vi "Constank Jerk Ref Mod (SubVI).vi"(0 "jav pos":dbl[](array[numeric])=[0.3, 0.2, 0.2], 1 "p_new":dbl[](array[numeric])=[2.0, 2.0, 0.0], 3 "Set point p":dbl[](array[numeric]), 4 "Eta":dbl[](array[numeric]), 5 "jav rad":dbl[](array[numeric])=[0.25, 0.15, 0.15], 7 "error in":errorcluster, 8 "Brake":bool, 9 "Set point theta":dbl[](array[numeric]), 10 "Go":bool, 12 "Go heading":bool, 13 "Theta_new":dbl[](array[numeric])=[0.0, 0.0, 45.0], 15 "time":dbl) -> (14 "javp":dbl[](array[numeric]), 16 "Eta des":dbl[](array[numeric]), 17 "Theta_ddot":dbl[](array[numeric]), 20 "Arrived":bool, 21 "Arrived yaw":bool, 23 "p_ddot":dbl[](array[numeric]), 24 "Nu des":dbl[](array[numeric]), 25 "Theta_d":dbl[](array[numeric]), 27 "error out":errorcluster)   [LabVIEW 2014, in "Guidance Library.lvlib" / "Constant Jerk Guidance.lvclass"]
uses:
  Constant Jerk Guidance.lvclass
  <vilib>/imath/engines/lvmath2/RunTimeEngine/BuiltInFunctions/rem/NIMS_rem_no checks.vi
  <instcachedir>/0/NIMS_rem_no checks_4BA74C9509D7485B8AB3E4C2ACC5A763.lvgen/NIMS_rem_no checks_4BA74C9509D7485B8AB3E4C2ACC5A763_000.vi
  <vilib>/imath/engines/lvmath2/RunTimeEngine/BuiltInFunctions/abs/NIMS_abs(signed).vi
  <instcachedir>/0/NIMS_abs(signed)_C4FCB8E6058B49B797C7C8D53CA5F6EC.lvgen/NIMS_abs(signed)_C4FCB8E6058B49B797C7C8D53CA5F6EC_000.vi
  <vilib>/imath/engines/lvmath2/RunTimeEngine/VariableToken/NIMS_VariableToken_CondDefined.vi
  <instcachedir>/0/NIMS_VariableToken_CondDefined_EE8DD211A89249938CE6537267F5C9B3.lvgen/NIMS_VariableToken_CondDefined_EE8DD211A89249938CE6537267F5C9B3_004.vi
  <vilib>/imathl/engines/lvmath/Functions/Error Handling/Create Error.vi
  <vilib>/imath/engines/lvmath2/RunTimeEngine/NodeEndStatement/NIMS_NodeEndStatement_Output.vi
  <instcachedir>/0/NIMS_NodeEndStatement_Output_53EC0D466D134D7ABD903AC30B43404B.lvgen/NIMS_NodeEndStatement_Output_53EC0D466D134D7ABD903AC30B43404B_001.vi
  <vilib>/imath/engines/lvmath2/RunTimeEngine/ErrorHandling/NIMS_Finalize Error.vi
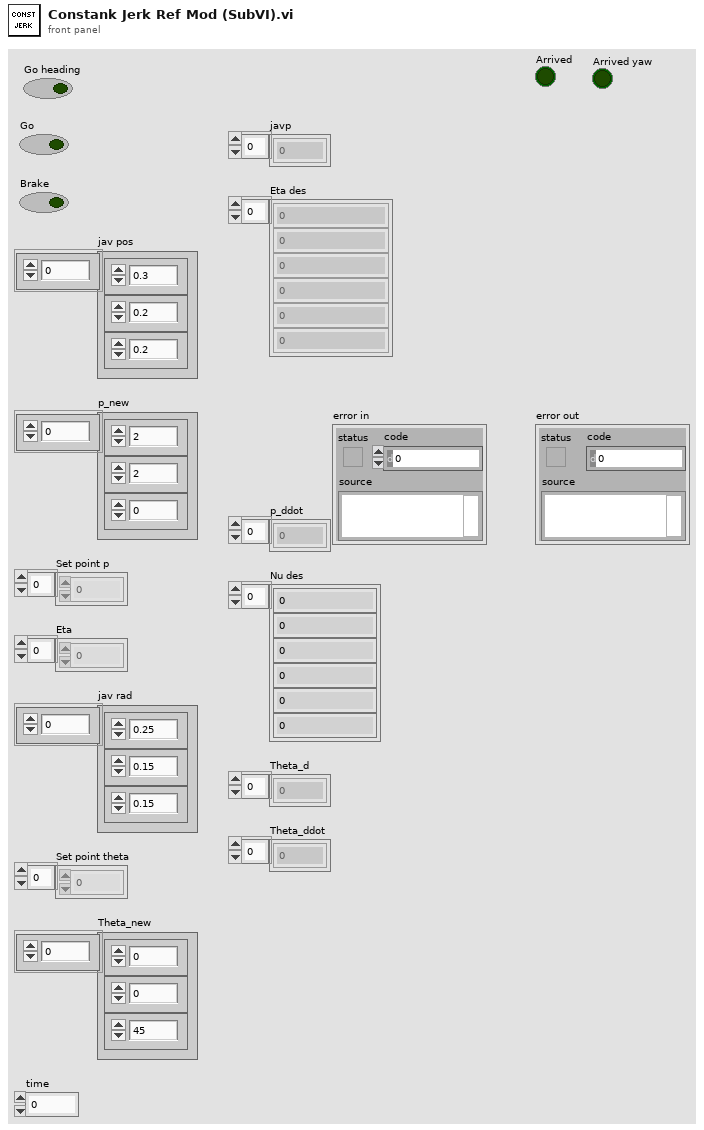
[diagram p1: front panel]
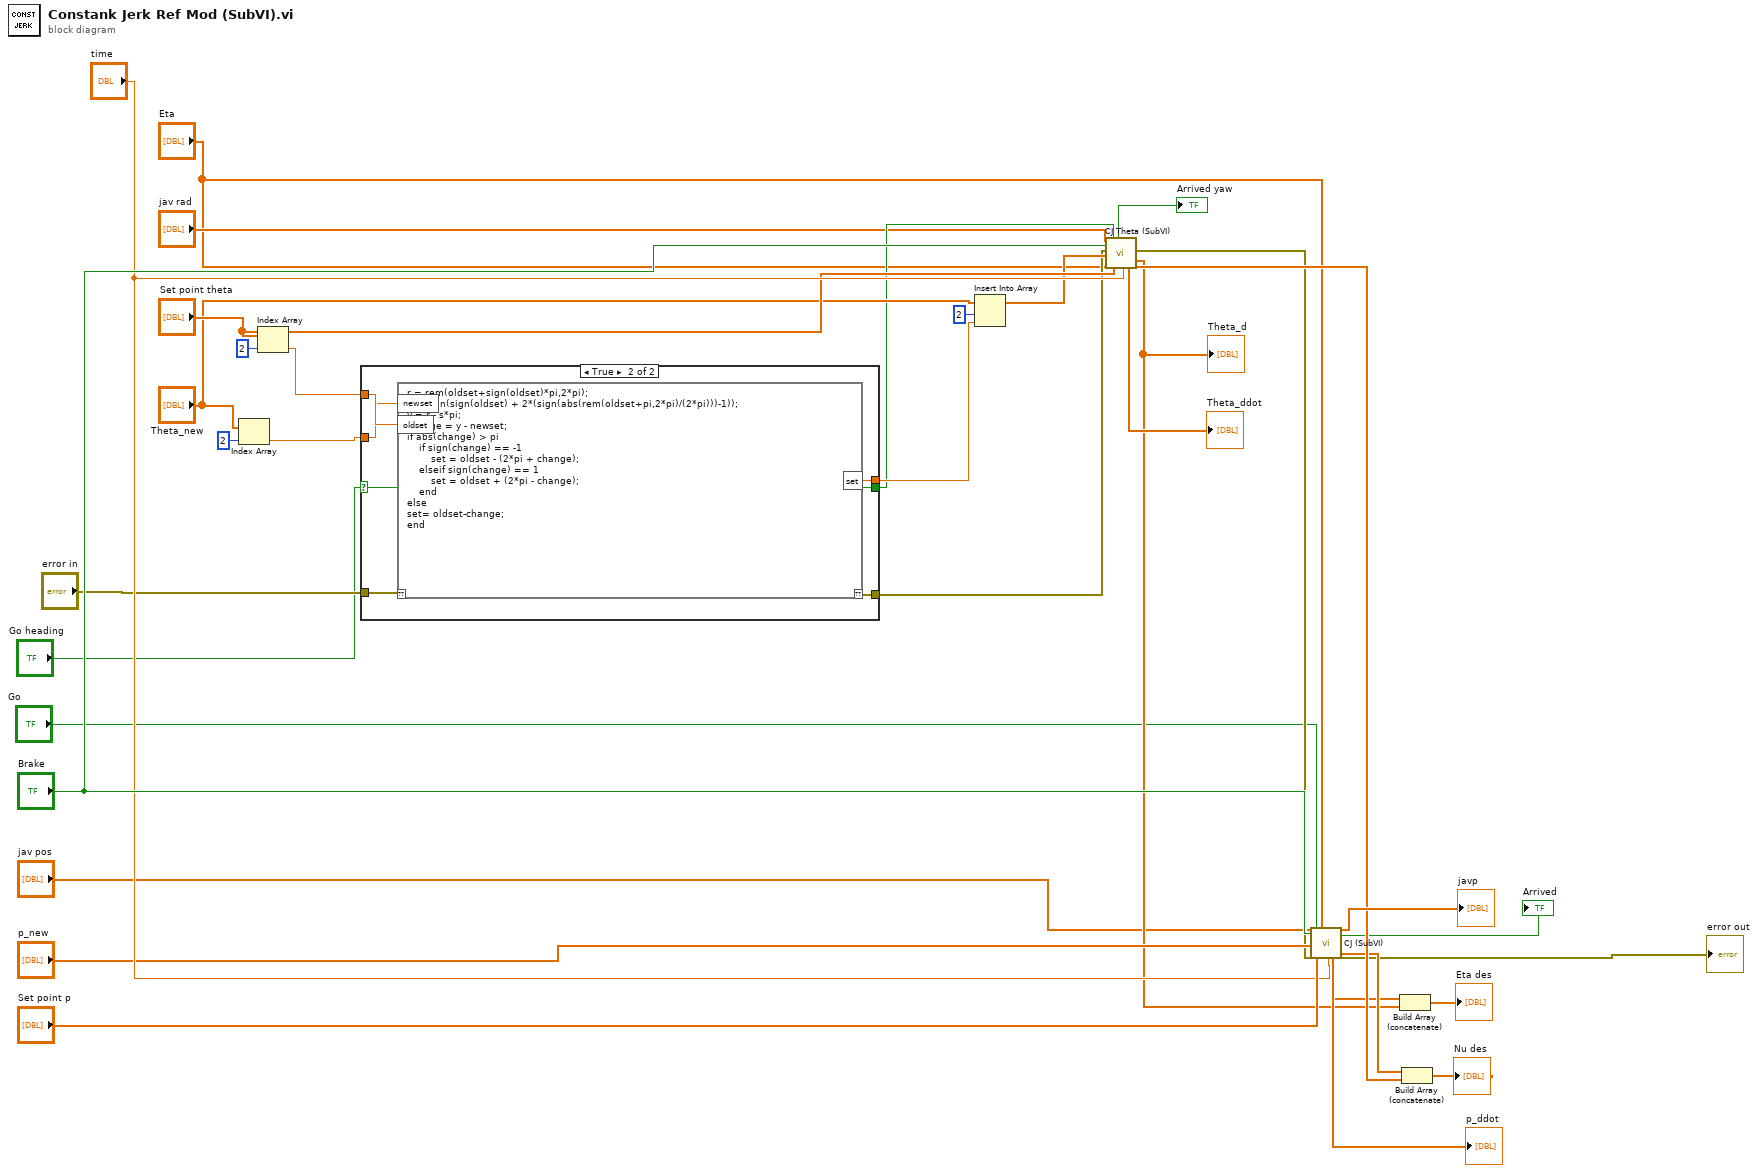
[diagram p0: block diagram]
diagram:
  n1 = Index Array(array="Theta_new", index=2) -> (element=w18:dbl)
  n2 = Index Array(array="Set point theta", index=2) -> (element=w20:dbl)
  n3 = case shown="True" "Go heading" {
    selector: "Go heading" -> [w35 w38]
    tunnel: w20 -> [_ w43]
    tunnel: w18 -> [w37 w42]
    tunnel: [w37 w41] -> w17
    tunnel: "error in" -> [w36 w40]
    tunnel: [w36 w39] -> w7
    tunnel: [w35 w38] -> w6
    frame False {
    }
    frame True {
      n4 = mathscript code="r = rem(oldset+sign(oldset)*pi,2*pi);\ns = sign(sign(oldset) + 2*(sign(abs(rem(oldset+pi,2*pi)/(2*pi)))-1));\ny = r - s*pi;\nchange = y - newset;\nif abs(change) > pi\n    if sign(change) == -1\n        set = oldset - (2*pi + change);\n    elseif sign(change) == 1\n        set = oldset + (2*pi - change);\n    end\nelse\nset= oldset-change;\nend"("??"=w40, "newset"=w42, "oldset"=w43) -> ("??"=w39:errorcluster, "set"=w41:dbl)
    }
  }
  n5 = Insert Into Array(array="Theta_new", index=2, new element=w17) -> (w14:dbl[])
  n6 = call "CJ Theta (SubVI).vi"("jav rad"="jav rad", "Brake"="Brake", "error in"=w7, "p_new"=w14, "Eta"="Eta", "Go"=w6, "p_old"="Set point theta", "time"="time") -> ("Arrived"=→"Arrived yaw":bool, "Theta_ddot"=→"Theta_ddot":dbl[], "error out"=w11:errorcluster, "Theta_d"=w9:dbl[], "omega"=w32:dbl[])  [unwired: 3 in, 4 out]
  "Theta_d" <- w9
  n7 = call "CJ (SubVI).vi"("jav pos"="jav pos", "Brake"="Brake", "p_new"="p_new", "error in"=w11, "Go"="Go", "p_old"="Set point p", "Eta"="Eta", "time"="time") -> ("Arrived"=→"Arrived":bool, "p_ddot"=→"p_ddot":dbl[], "javp"=→"javp":dbl[], "p_d"=w26:dbl[], "nu_d"=w31:dbl[], "error out"=→"error out":errorcluster)  [unwired: 14 in]
  n8 = Build Array (concatenate)(w26, w9) -> (→"Eta des":dbl[])
  n9 = Build Array (concatenate)(w31, w32) -> (→"Nu des":dbl[])
